vi "URL_to_Variable.vi"(11 "URL":string="\\\\HousesOfTheHoly\\Leiden MNK\\Leiden MNK Front Panel\\MNK MF P_low") -> (3 "Name":string)   [LabVIEW 2016]
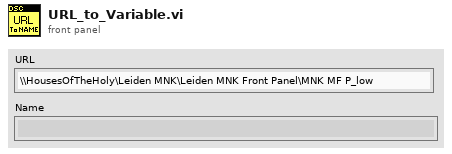
[diagram p1: front panel]
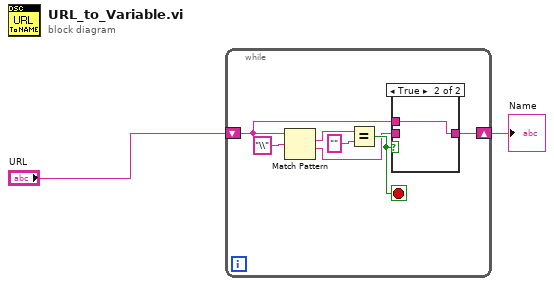
[diagram p0: block diagram]
diagram:
  n1 = while {
    shift-right: [w5] -> w1
    shift-left: "URL" -> [w3]
    stop <- w6 stop-if-true
    n2 = Match Pattern(string=w3, regular expression="\\") -> (match substring=w8:string, after substring=w4:string)  [unwired: 1 in, 2 out]
    n3 = Equal?(x=w8, y="" ("regular expression")) -> (x = y?=w6:bool)
    n4 = case shown="True" w6 {
      tunnel: [w10 w11] -> w5
      tunnel: w4 -> [w10 _]
      tunnel: w3 -> [_ w11]
      frame False {
      }
      frame True {
      }
    }
  }
  "Name" <- w1
